vi "FiberMRI_Main_NI.vi"() -> ()   [LabVIEW 2010]
doc: "Acquisition software for combined single-photon fluorescence and fMRI experiments."
uses:
  typedefs/storage_parameters_cluster.ctl
  typedefs/experiment_mode_enum.ctl
  typedefs/stimulation_parameters.ctl
  typedefs/acquisition_parameters_NI_cluster.ctl
  typedefs/main_state_enum.ctl
  typedefs/control_daq_enum.ctl
  typedefs/control_display_enum.ctl
  typedefs/control_storage_enum.ctl
  typedefs/control_analysis_enum.ctl
  <vilib>/Utility/error.llb/DialogType.ctl
  typedefs/control_stim_enum.ctl
  typedefs/all_frontpanel_parameters_NI.ctl
  <vilib>/DAQmx/write.llb/DAQmx Write (Digital Bool 1Line 1Point).vi
  <vilib>/DAQmx/create/channels.llb/DAQmx Create Channel (DO-Digital Output).vi
  <vilib>/daqmx/miscellaneous.llb/DAQmx Fill In Error Info.vi
  globals/exit.vi
panel:
  in  "Acquisition parameters":T1={"Physical channels"="", "Shutter line"="", "Triggered?"=FALSE, "Sample rate"=1000.0, "Pixels to integrate"=10, "Effective data rate"=0.0, "Read chunk size"=100, "Samples to read"=2000, "Run mode"=enum."Continuously"} {"Pixels to integrate" min=1 step=1; "Sample rate" min=10.0 max=25000.0}
  out "Running":bool
  in  "Stimulation parameters":T2={"Physical channel"="Dev0/1stPortB/Do0", "Write chunk size"=1, "Sample rate"=1.0, "Stim onset"=0.0, "Stim frequency"=1.0, "ON time"=40.0, "OFF time"=120.0, "Repetitions"=1.0} {"Write chunk size" min=100 max=100000; "Sample rate" min=10.0 max=10000.0; "Repetitions" min=0.0 max=10.0 step=1.0; "OFF time" min=0.0 max=1000.0; "ON time" min=0.0 max=1000.0; "Stim onset" min=0.0 max=100.0; "Stim frequency" min=1.0 max=40.0 step=1.0}
  in  "Reset":bool
  in  "Shutter":bool
  in  "Experiment mode":T3
  in  "Storage parameters":T4
  in  "Run":bool
  in  "Quit":bool
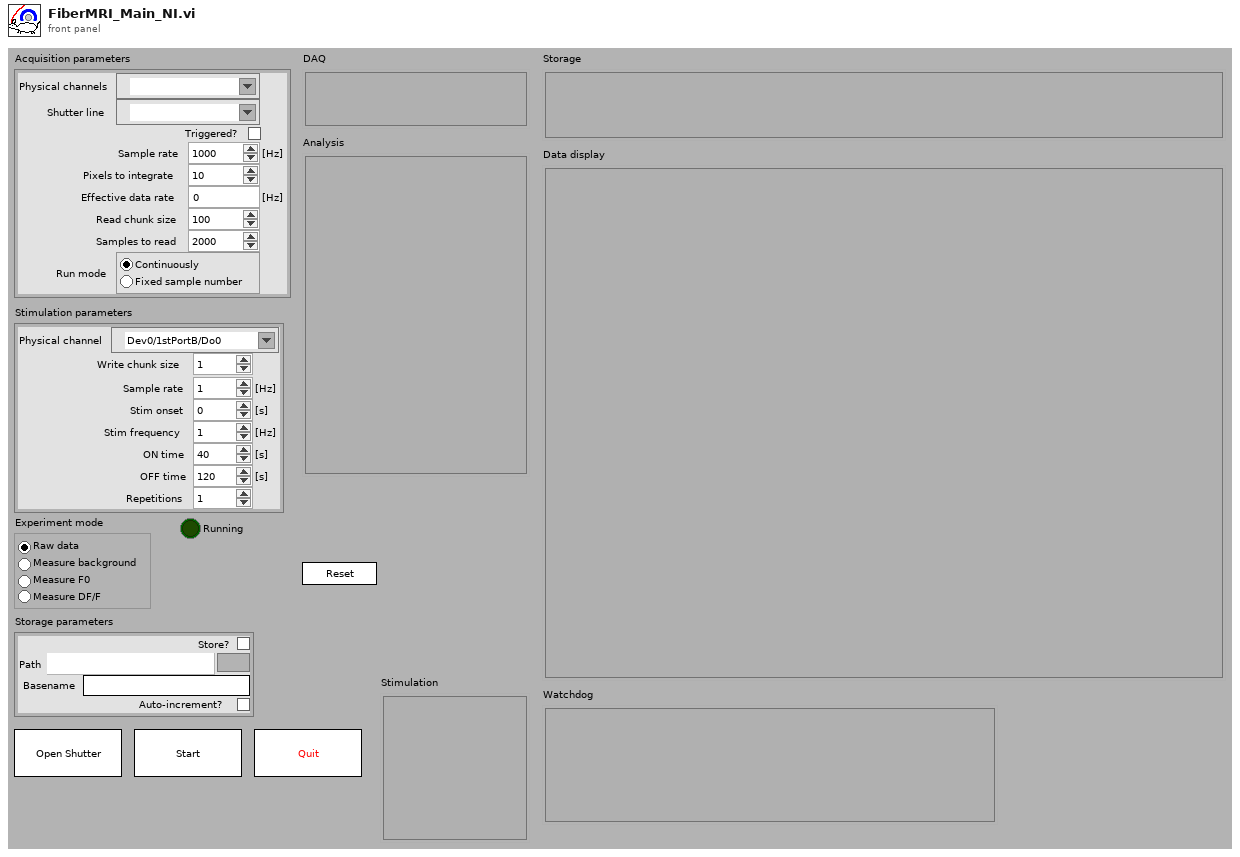
[diagram p1: front panel]
types:
  T1 = typedef "acquisition_parameters_NI_cluster.ctl" = cluster{"Physical channels":tag, "Shutter line":tag, "Triggered?":bool, "Sample rate":dbl, "Pixels to integrate":i32, "Effective data rate":dbl, "Read chunk size":i32, "Samples to read":i32, "Run mode":enum32{"Continuously", "Fixed sample number"}}
  T2 = typedef "stimulation_parameters.ctl" = cluster{"Physical channel":tag, "Write chunk size":i32, "Sample rate":dbl, "Stim onset":dbl, "Stim frequency":dbl, "ON time":dbl, "OFF time":dbl, "Repetitions":dbl}
  T3 = typedef "experiment_mode_enum.ctl" = enum32{"Raw data", "Measure background", "Measure F0", "Measure DF/F"}
  T4 = typedef "storage_parameters_cluster.ctl" = cluster{"Store?":bool, "Path":path, "Basename":string, "Auto-increment?":bool}
  T5 = typedef "all_frontpanel_parameters_NI.ctl" = cluster{"Acquisition parameters":T1, "Stimulation parameters":T2, "Experiment mode":T3, "Storage parameters":T4}
  T6 = typedef "DialogType.ctl" = u16
  T7 = typedef "main_state_enum.ctl" = enum16{"Init", "ParamsChanged", "Start", "Stop", "SetShutter", "Reset", "Save", "Quit"}
  T8 = cluster{"Control_DAQ_Queue":refnum<queue>, "Control_Storage_Queue":refnum<queue>, "Control_Display_Queue":refnum<queue>, "Control_Analysis_Queue":refnum<queue>, "Control_Stim_Queue":refnum<queue>}
  T9 = typedef "control_stim_enum.ctl" = enum16{"Init", "Stim", "Stop", "Quit"}
  T10 = cluster{"Control stim Enum":T9, "variant":variant}
  T11 = typedef "control_analysis_enum.ctl" = enum16{"Init", "Analyze", "Reset", "Stop", "Quit"}
  T12 = cluster{"Control Analysis Enum":T11, "variant":variant}
  T13 = typedef "control_display_enum.ctl" = enum16{"Init", "Display", "Quit"}
  T14 = cluster{"Control display enum":T13, "variant":variant}
  T15 = typedef "control_storage_enum.ctl" = enum16{"Init", "Discard", "Store", "Reset", "Stop", "Quit"}
  T16 = cluster{"Control storage enum":T15, "variant":variant}
  T17 = typedef "control_daq_enum.ctl" = enum16{"Init", "GetCont", "GetNoSamples", "Stop", "Quit"}
  T18 = cluster{"Control DAQ Enum":T17, "variant":variant}
  T19 = cluster{"Acquisition parameters":T1, "Stimulation parameters":T2}
  T20 = cluster{"Control DAQ Enum":T17, "Variant":variant}
  T21 = cluster{"Experiment mode":T3, "Pixels to integrate":i32, "#channels":i32, "Iteration":i32}
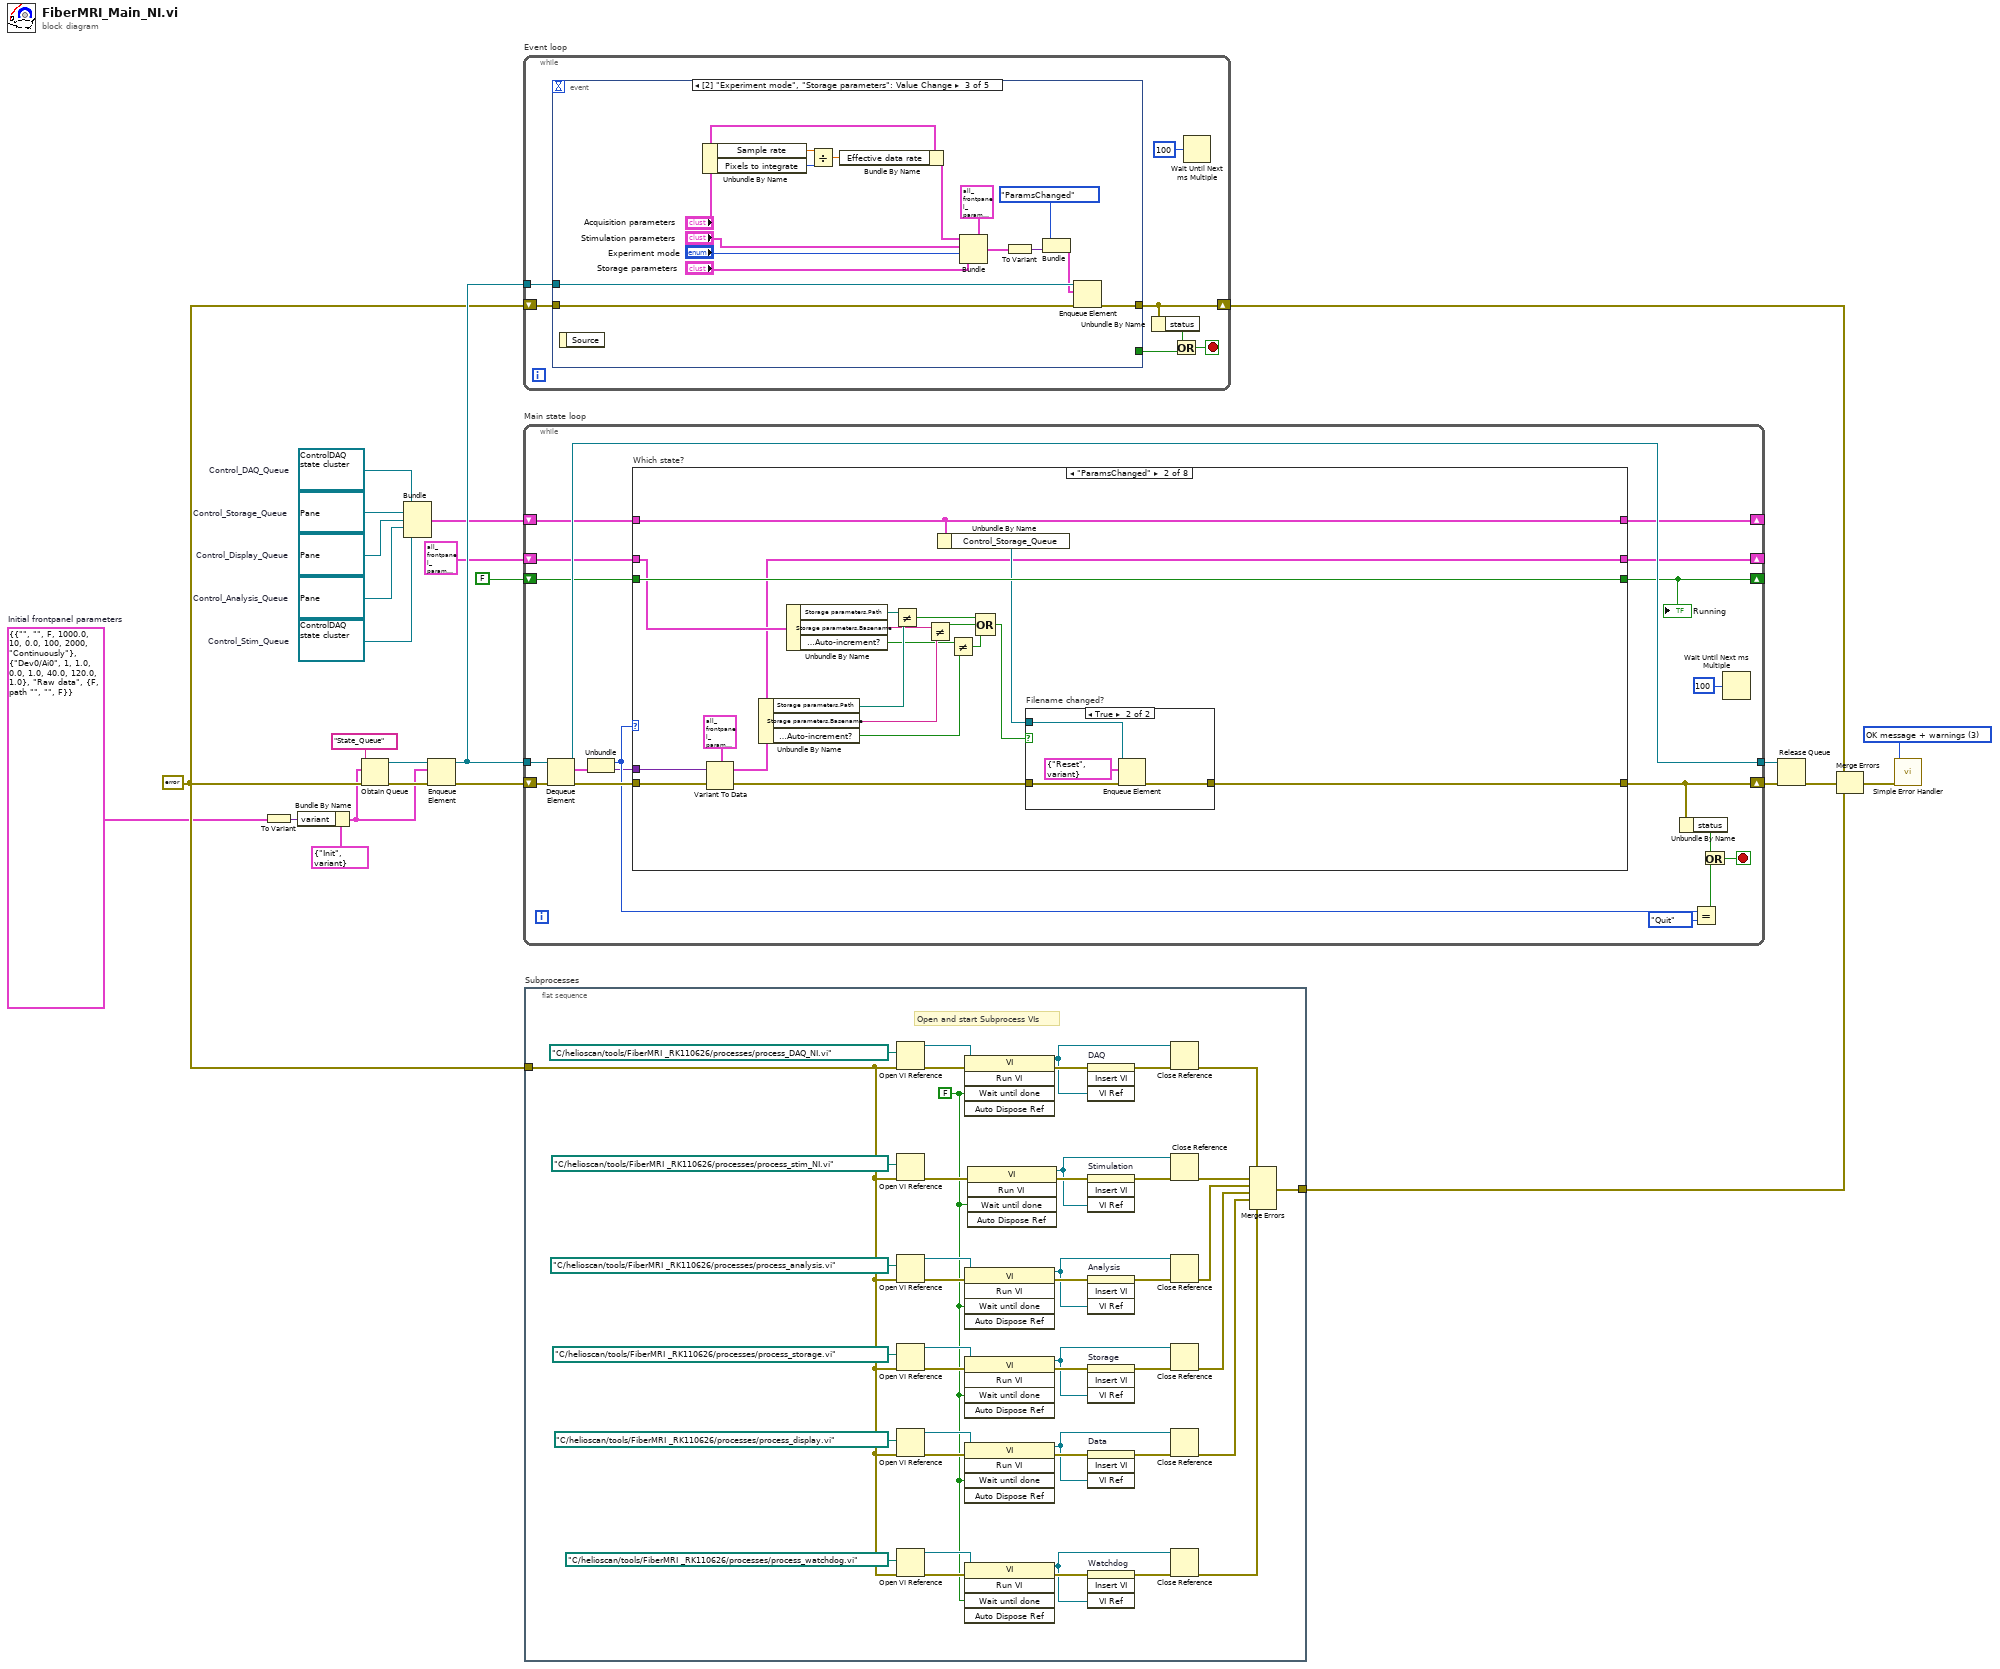
[diagram p0: block diagram]
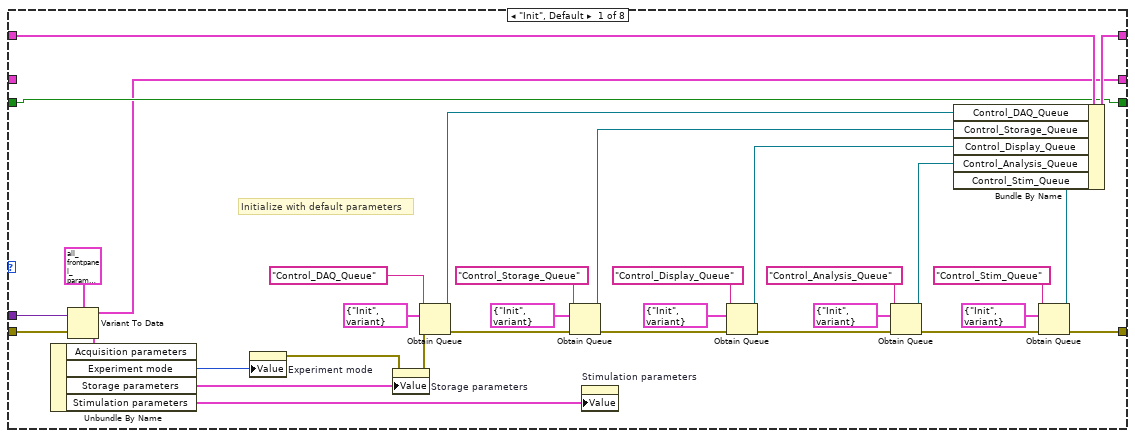
[diagram p2: hidden frame]
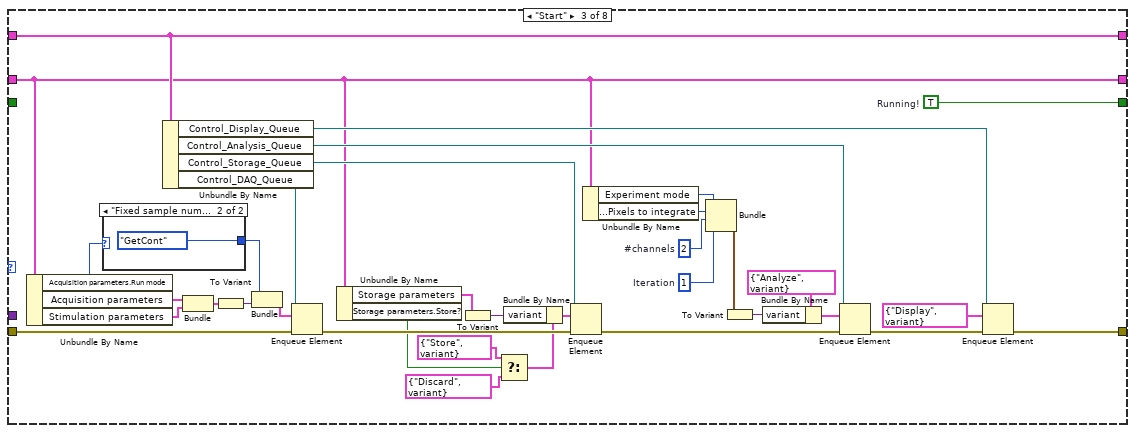
[diagram p4: hidden frame]
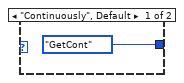
[diagram p5: hidden frame]
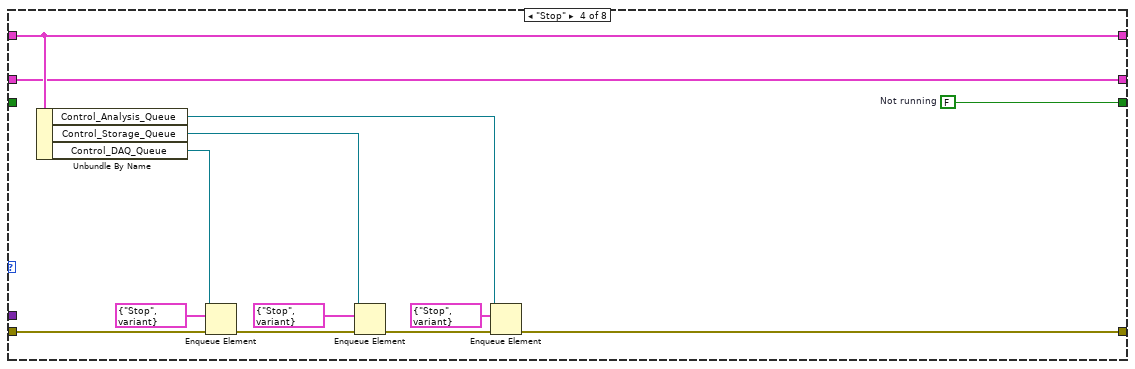
[diagram p6: hidden frame]
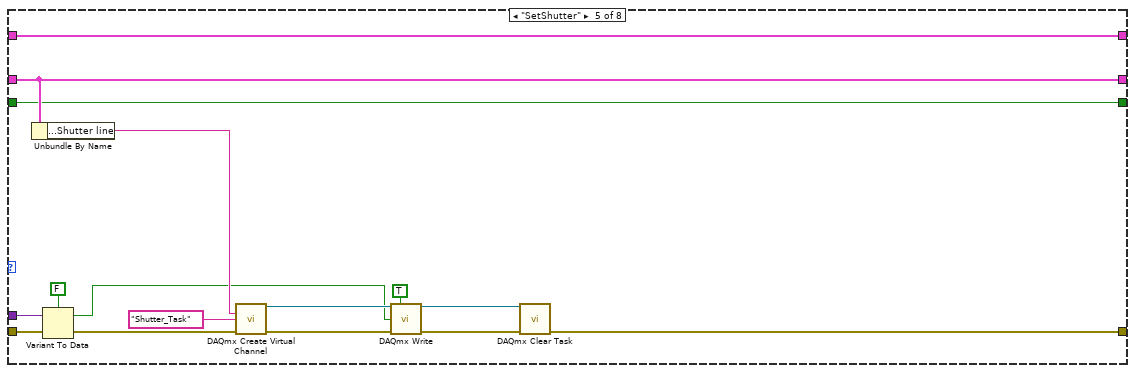
[diagram p7: hidden frame]
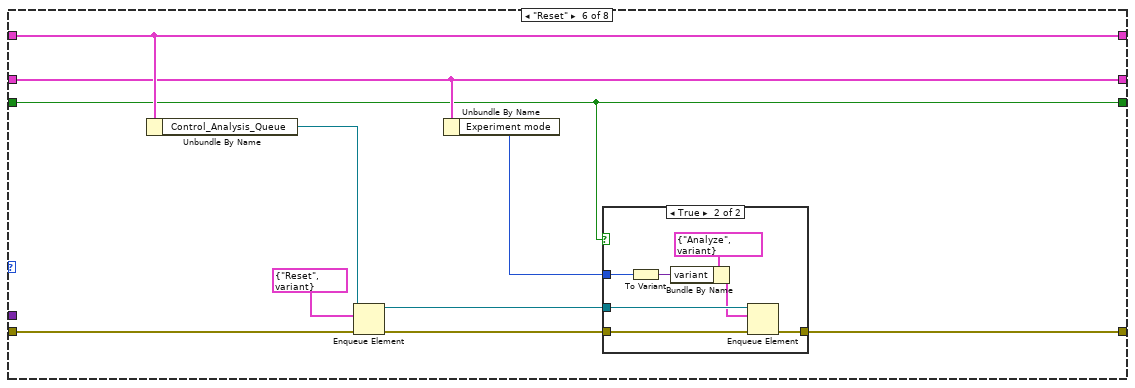
[diagram p8: hidden frame]
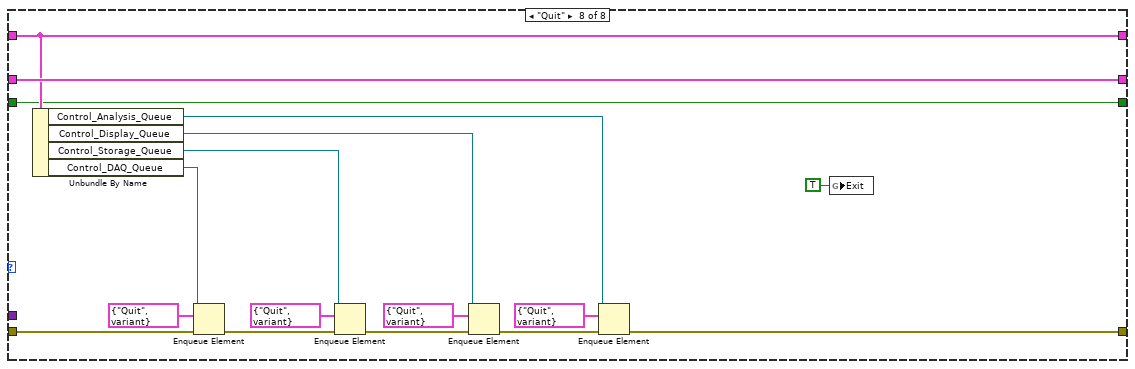
[diagram p11: hidden frame]
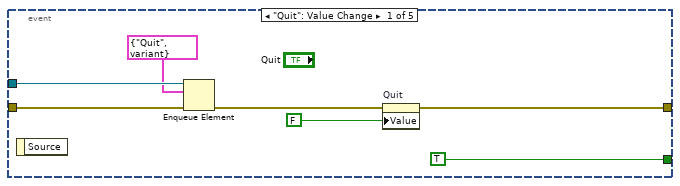
[diagram p12: hidden frame]
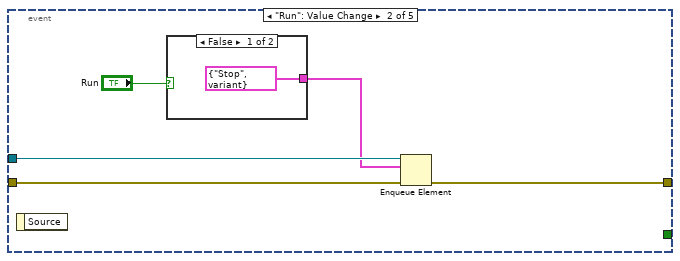
[diagram p13: hidden frame]
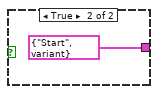
[diagram p14: hidden frame]
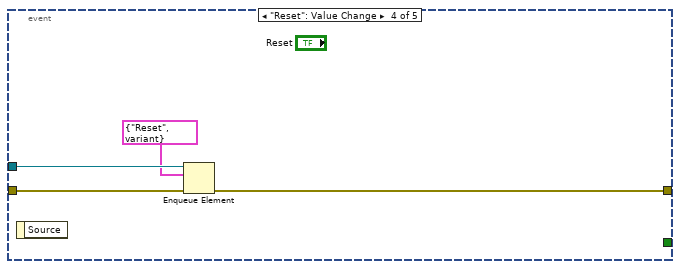
[diagram p15: hidden frame]
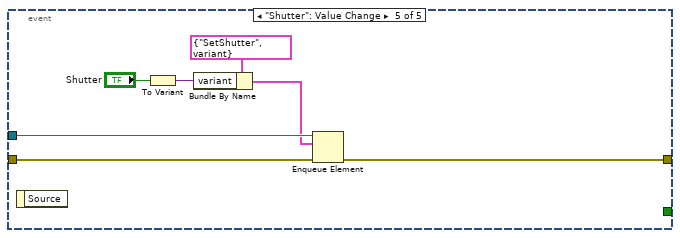
[diagram p16: hidden frame]
diagram:
  w2 = T5 {"Acquisition parameters"={"Physical channels"="", "Shutter line"="", "Triggered?"=FALSE, "Sample rate"=1000.0, "Pixels to integrate"=10, "Effective data rate"=0.0, "Read chunk size"=100, "Samples to read"=2000, "Run mode"=enum."Continuously"}, "Stimulation parameters"={"Physical channel"="Dev0/Ai0", "Write chunk size"=1, "Sample rate"=1.0, "Stim onset"=0.0, "Stim frequency"=1.0, "ON time"=40.0, "OFF time"=120.0, "Repetitions"=1.0}, "Experiment mode"=enum."Raw data", "Storage parameters"={"Store?"=FALSE, "Path"=path "", "Basename"="", "Auto-increment?"=FALSE}}  # Initial frontpanel parameters
  w3 = refnum<queue> refnum  # Control_Stim_Queue
  w13 = T6 3 items=["no dialog", "OK message", "continue or stop message", "OK message + warnings", "continue/stop + warnings"] ("type of dialog (OK msg:1)")
  w14 = refnum<queue> refnum  # Control_Analysis_Queue
  w15 = refnum<queue> refnum  # Control_Storage_Queue
  w16 = refnum<queue> refnum  # Control_Display_Queue
  w10 = errorcluster {"status"=FALSE, "code"=0, "source"=""} ("error out")
  w19 = refnum<queue> refnum  # Control_DAQ_Queue
  n1 = To Variant(anything=w2) -> (Variant=w5:variant)
  n2 = Bundle By Name(cluster=cluster{"State Enum":T7, "variant":variant} {"State Enum"=enum."Init", "variant"=variant}, "variant"=w5) -> (w4:cluster{"State Enum":T7, "variant":variant})
  n3 = Obtain Queue(name (unnamed)="State_Queue", element data type=w4, error in (no error)=w10) -> (queue out=w24:refnum<queue>, error out=w22:errorcluster)  [unwired: 2 in, 1 out]
  n4 = Bundle("Control_DAQ_Queue"=w19, "Control_Storage_Queue"=w15, "Control_Display_Queue"=w16, "Control_Analysis_Queue"=w14, "Control_Stim_Queue"=w3) -> (w18:T8)  [unwired: 1 in]
  n5 = Enqueue Element(queue=w24, element=w4, error in (no error)=w22) -> (queue out=w23:refnum<queue>, error out=w17:errorcluster)  [unwired: 1 in, 1 out]
  n6 = while "Event loop" {
    shift-right: [w28] -> w11
    shift-left: w10 -> [w31]
    tunnel: w23 -> [w32]
    stop <- w29 stop-if-true
    n7 = event shown="[2] \"Experiment mode\", \"Storage parameters\": Value Change" {
      selector: _ -> [_ _ _ _ _]
      dyn-events: _ -> [_ _ _ _ _]
      timeout: _ -> [_ _ _ _ _]
      tunnel: w32 -> [w38 w43 w62 w65 w72]
      tunnel: w31 -> [w39 w42 w47 w66 w73]
      tunnel: [w34 w40 w54 w64 w67] -> w28
      tunnel: [TRUE _ _ _ _] -> w30
      event "Quit": Value Change {
        n8 = event-data() -> ()  [unwired: 1 in, 1 out]
        n9 = Enqueue Element(queue=w38, element=cluster{"State Enum":T7, "variant":variant} {"State Enum"=enum."Quit", "variant"=variant}, error in (no error)=w39) -> (error out=w35:errorcluster)  [unwired: 1 in, 2 out]
        n10 = property on="Quit" class="Bool (strict)"(error in=w35, "Value"=FALSE) -> (error out=w34:errorcluster)  [unwired: 1 in, 1 out]
      }
      event "Run": Value Change {
        n11 = event-data() -> ()  [unwired: 1 in, 1 out]
        n12 = case shown="False" "Run" {
          tunnel: [cluster{"State Enum":T7, "variant":variant} {"State Enum"=enum."Stop", "variant"=variant} cluster{"State Enum":T7, "variant":variant} {"State Enum"=enum."Start", "variant"=variant}] -> w41
          frame False {
          }
          frame True {
          }
        }
        n13 = Enqueue Element(queue=w43, element=w41, error in (no error)=w42) -> (error out=w40:errorcluster)  [unwired: 1 in, 2 out]
      }
      event Value Change {
        n14 = event-data() -> ()  [unwired: 1 in, 1 out]
        n15 = Unbundle By Name("Acquisition parameters") -> ("Sample rate"=w56:dbl, "Pixels to integrate"=w57:i32)
        n16 = Divide(x=w56, y=w57) -> (x/y=w55:dbl)
        n17 = Bundle By Name(cluster="Acquisition parameters", "Effective data rate"=w55) -> (w53:T1)
        n18 = Bundle(cluster=T5 {"Acquisition parameters"={"Physical channels"="", "Shutter line"="", "Triggered?"=FALSE, "Sample rate"=1000.0, "Pixels to integrate"=10, "Effective data rate"=0.0, "Read chunk size"=100, "Samples to read"=2000, "Run mode"=enum."Continuously"}, "Stimulation parameters"={"Physical channel"="Dev0/Ai0", "Write chunk size"=1, "Sample rate"=1.0, "Stim onset"=0.0, "Stim frequency"=1.0, "ON time"=40.0, "OFF time"=120.0, "Repetitions"=1.0}, "Experiment mode"=enum."Raw data", "Storage parameters"={"Store?"=FALSE, "Path"=path "", "Basename"="", "Auto-increment?"=FALSE}} ("All frontpanel parameters"), "Acquisition parameters"=w53, "Stimulation parameters"="Stimulation parameters", "Experiment mode"="Experiment mode", "Storage parameters"="Storage parameters") -> (w58:T5)
        n19 = To Variant(anything=w58) -> (Variant=w61:variant)
        n20 = Bundle("State Enum"=main_state_enum."ParamsChanged", "Variant"=w61) -> (w59:cluster{"State Enum":T7, "Variant":variant})  [unwired: 1 in]
        n21 = Enqueue Element(queue=w62, element=w59, error in (no error)=w47) -> (error out=w54:errorcluster)  [unwired: 1 in, 2 out]
      }
      event "Reset": Value Change {
        n22 = event-data() -> ()  [unwired: 1 in, 1 out]
        n23 = Enqueue Element(queue=w65, element=cluster{"State Enum":T7, "variant":variant} {"State Enum"=enum."Reset", "variant"=variant}, error in (no error)=w66) -> (error out=w64:errorcluster)  [unwired: 1 in, 2 out]
      }
      event "Shutter": Value Change {
        n24 = event-data() -> ()  [unwired: 1 in, 1 out]
        n25 = To Variant(anything="Shutter") -> (Variant=w70:variant)
        n26 = Bundle By Name(cluster=cluster{"State Enum":T7, "variant":variant} {"State Enum"=enum."SetShutter", "variant"=variant} ("element"), "variant"=w70) -> (w68:cluster{"State Enum":T7, "variant":variant})
        n27 = Enqueue Element(queue=w72, element=w68, error in (no error)=w73) -> (error out=w67:errorcluster)  [unwired: 1 in, 2 out]
      }
    }
    n28 = Unbundle By Name(w28) -> ("status"=w27:bool)
    n29 = Or(x=w27, y=w30) -> (x .or. y?=w29:bool)
    n30 = Wait Until Next ms Multiple(millisecond multiple=u32 100) -> ()  [unwired: 1 out]
  }
  n31 = while "Main state loop" {
    shift-right: [w80] -> w25
    shift-left: w17 -> [w90]
    shift-right: [w84] -> _
    shift-left: T5 {"Acquisition parameters"={"Physical channels"="", "Shutter line"="", "Triggered?"=FALSE, "Sample rate"=1000.0, "Pixels to integrate"=10, "Effective data rate"=0.0, "Read chunk size"=100, "Samples to read"=2000, "Run mode"=enum."Continuously"}, "Stimulation parameters"={"Physical channel"="Dev0/Ai0", "Write chunk size"=1, "Sample rate"=1.0, "Stim onset"=0.0, "Stim frequency"=1.0, "ON time"=40.0, "OFF time"=120.0, "Repetitions"=1.0}, "Experiment mode"=enum."Raw data", "Storage parameters"={"Store?"=FALSE, "Path"=path "", "Basename"="", "Auto-increment?"=FALSE}} ("Initial frontpanel parameters") -> [w83]
    tunnel: w23 -> [w92]
    tunnel: [w91] -> w21
    shift-right: [w81] -> _
    shift-left: w18 -> [w82]
    shift-right: [w75] -> _
    shift-left: FALSE -> [w76]
    stop <- w77 stop-if-true
    n32 = Dequeue Element(queue=w92, error in (no error)=w90) -> (queue out=w91:refnum<queue>, element=w87:cluster{"State Enum":T7, "variant":variant}, error out=w89:errorcluster)  [unwired: 1 in, 1 out]
    n33 = Unbundle(w87) -> ("State Enum"=w86:T7, "variant"=w85:variant)
    n34 = case "Which state?" shown="\"ParamsChanged\"" w86 {
      tunnel: w89 -> [w101 w143 w184 w199 w213 w224 w237 w254]
      tunnel: [w97 w127 w175 w189 w200 w219 w237 w242] -> w80
      tunnel: w85 -> [w99 w144 _ _ w212 _ _ _]
      tunnel: [w100 w126 w165 w188 w214 w221 w236 w253] -> w84
      tunnel: w83 -> [_ w141 w165 w188 w214 w221 w236 w253]
      tunnel: w82 -> [w120 w130 w179 w197 w215 w225 w235 w251]
      tunnel: [w119 w130 w179 w197 w215 w225 w235 w251] -> w81
      tunnel: w76 -> [w107 w142 _ _ w210 w216 w234 w239]
      tunnel: [w107 w142 w166 w187 w210 w216 w234 w239] -> w75
      frame "Init", Default {
        # "Initialize with default parameters"
        n35 = Variant To Data(error in=w101, Variant=w99, type=T5 {"Acquisition parameters"={"Physical channels"="", "Shutter line"="", "Triggered?"=FALSE, "Sample rate"=1000.0, "Pixels to integrate"=10, "Effective data rate"=0.0, "Read chunk size"=100, "Samples to read"=2000, "Run mode"=enum."Continuously"}, "Stimulation parameters"={"Physical channel"="Dev0/Ai0", "Write chunk size"=1, "Sample rate"=1.0, "Stim onset"=0.0, "Stim frequency"=1.0, "ON time"=40.0, "OFF time"=120.0, "Repetitions"=1.0}, "Experiment mode"=enum."Raw data", "Storage parameters"={"Store?"=FALSE, "Path"=path "", "Basename"="", "Auto-increment?"=FALSE}} ("Initial frontpanel parameters")) -> (data=w100:T5)  [unwired: 1 out]
        n36 = Unbundle By Name(w100) -> ("Experiment mode"=w106:T3, "Storage parameters"=w103:T4, "Stimulation parameters"=w102:T2)  [unwired: 1 out]
        n37 = property on="Experiment mode" class="RadioBtnsControl (strict)"("Value"=w106) -> (error out=w105:errorcluster)  [unwired: 2 in, 1 out]
        n38 = property on="Storage parameters" class="Clust (strict)"(error in=w105, "Value"=w103) -> (error out=w104:errorcluster)  [unwired: 1 in, 1 out]
        n39 = Obtain Queue(name (unnamed)="Control_DAQ_Queue", element data type=T18 {"Control DAQ Enum"=enum."Init", "variant"=variant} ("ControlDAQ state cluster"), error in (no error)=w104) -> (queue out=w118:refnum<queue>, error out=w116:errorcluster)  [unwired: 2 in, 1 out]
        n40 = Obtain Queue(name (unnamed)="Control_Storage_Queue", element data type=T16 {"Control storage enum"=enum."Init", "variant"=variant}, error in (no error)=w116) -> (queue out=w117:refnum<queue>, error out=w115:errorcluster)  [unwired: 2 in, 1 out]
        n41 = property on="Stimulation parameters" class="Clust (strict)"("Value"=w102) -> ()  [unwired: 2 in, 2 out]
        n42 = Obtain Queue(name (unnamed)="Control_Display_Queue", element data type=T14 {"Control display enum"=enum."Init", "variant"=variant}, error in (no error)=w115) -> (queue out=w112:refnum<queue>, error out=w111:errorcluster)  [unwired: 2 in, 1 out]
        n43 = Obtain Queue(name (unnamed)="Control_Analysis_Queue", element data type=T12 {"Control Analysis Enum"=enum."Init", "variant"=variant}, error in (no error)=w111) -> (queue out=w108:refnum<queue>, error out=w98:errorcluster)  [unwired: 2 in, 1 out]
        n44 = Obtain Queue(name (unnamed)="Control_Stim_Queue", element data type=T10 {"Control stim Enum"=enum."Init", "variant"=variant} ("ControlDAQ state cluster"), error in (no error)=w98) -> (queue out=w94:refnum<queue>, error out=w97:errorcluster)  [unwired: 2 in, 1 out]
        n45 = Bundle By Name(cluster=w120, "Control_DAQ_Queue"=w118, "Control_Storage_Queue"=w117, "Control_Display_Queue"=w112, "Control_Analysis_Queue"=w108, "Control_Stim_Queue"=w94) -> (w119:T8)
      }
      frame "ParamsChanged" {
        n46 = Variant To Data(error in=w143, Variant=w144, type=T5 {"Acquisition parameters"={"Physical channels"="", "Shutter line"="", "Triggered?"=FALSE, "Sample rate"=1000.0, "Pixels to integrate"=10, "Effective data rate"=0.0, "Read chunk size"=100, "Samples to read"=2000, "Run mode"=enum."Continuously"}, "Stimulation parameters"={"Physical channel"="Dev0/Ai0", "Write chunk size"=1, "Sample rate"=1.0, "Stim onset"=0.0, "Stim frequency"=1.0, "ON time"=40.0, "OFF time"=120.0, "Repetitions"=1.0}, "Experiment mode"=enum."Raw data", "Storage parameters"={"Store?"=FALSE, "Path"=path "", "Basename"="", "Auto-increment?"=FALSE}} ("Initial frontpanel parameters")) -> (error out=w128:errorcluster, data=w126:T5)
        n47 = Unbundle By Name(w126) -> ("Storage parameters.Path"=w139:path, "Storage parameters.Basename"=w137:string, "Storage parameters.Auto-increment?"=w135:bool)
        n48 = Unbundle By Name(w141) -> ("Storage parameters.Path"=w140:path, "Storage parameters.Basename"=w138:string, "Storage parameters.Auto-increment?"=w136:bool)
        n49 = Not Equal?(x=w140, y=w139) -> (x != y?=w134:bool)
        n50 = Not Equal?(x=w138, y=w137) -> (x != y?=w133:bool)
        n51 = Unbundle By Name(w130) -> ("Control_Storage_Queue"=w129:refnum<queue>)
        n52 = Not Equal?(x=w136, y=w135) -> (x != y?=w132:bool)
        n53 = Compound Arithmetic op=OR(w134, w133, w132) -> (w131:bool)
        n54 = case "Filename changed?" shown="True" w131 {
          tunnel: w129 -> [_ w149]
          tunnel: w128 -> [w145 w147]
          tunnel: [w145 w146] -> w127
          frame False {
          }
          frame True {
            n55 = Enqueue Element(queue=w149, element=T16 {"Control storage enum"=enum."Reset", "variant"=variant}, error in (no error)=w147) -> (error out=w146:errorcluster)  [unwired: 1 in, 2 out]
          }
        }
      }
      frame "Start" {
        w150 = 1  # Iteration
        w151 = 2  # #channels
        w166 = TRUE  # Running!
        n56 = Unbundle By Name(w165) -> ("Acquisition parameters.Run mode"=w181:enum32{"Continuously", "Fixed sample number"}, "Acquisition parameters"=w160:T1, "Stimulation parameters"=w159:T2)
        n57 = case shown="\"Fixed sample number\"" w181 {
          tunnel: [control_daq_enum."GetCont" ("Control DAQ Enum") control_daq_enum."GetCont" ("Control DAQ Enum")] -> w180
          frame "Continuously", Default {
          }
          frame "Fixed sample number" {
          }
        }
        n58 = Unbundle By Name(w179) -> ("Control_Display_Queue"=w173:refnum<queue>, "Control_Analysis_Queue"=w170:refnum<queue>, "Control_Storage_Queue"=w176:refnum<queue>, "Control_DAQ_Queue"=w178:refnum<queue>)
        n59 = Bundle("Acquisition parameters"=w160, "Stimulation parameters"=w159) -> (w158:T19)  [unwired: 1 in]
        n60 = To Variant(anything=w158) -> (Variant=w183:variant)
        n61 = Bundle("Control DAQ Enum"=w180, "Variant"=w183) -> (w182:T20)  [unwired: 1 in]
        n62 = Enqueue Element(queue=w178, element=w182, error in (no error)=w184) -> (error out=w177:errorcluster)  [unwired: 1 in, 2 out]
        n63 = Unbundle By Name(w165) -> ("Storage parameters"=w161:T4, "Storage parameters.Store?"=w156:bool)
        n64 = To Variant(anything=w161) -> (Variant=w157:variant)
        n65 = Select(t=T16 {"Control storage enum"=enum."Store", "variant"=variant} ("element"), s=w156, f=T16 {"Control storage enum"=enum."Discard", "variant"=variant} ("element")) -> (s? t:f=w153:T16)
        n66 = Bundle By Name(cluster=w153, "variant"=w157) -> (w152:T16)
        n67 = Enqueue Element(queue=w176, element=w152, error in (no error)=w177) -> (error out=w172:errorcluster)  [unwired: 1 in, 2 out]
        n68 = Unbundle By Name(w165) -> ("Experiment mode"=w164:T3, "Acquisition parameters.Pixels to integrate"=w163:i32)
        n69 = Bundle("Experiment mode"=w164, "Pixels to integrate"=w163, "#channels"=w151, "Iteration"=w150) -> (w162:T21)  [unwired: 1 in]
        n70 = To Variant(anything=w162) -> (Variant=w169:variant)
        n71 = Bundle By Name(cluster=T12 {"Control Analysis Enum"=enum."Analyze", "variant"=variant} ("element"), "variant"=w169) -> (w167:T12)
        n72 = Enqueue Element(queue=w170, element=w167, error in (no error)=w172) -> (error out=w171:errorcluster)  [unwired: 1 in, 2 out]
        n73 = Enqueue Element(queue=w173, element=T14 {"Control display enum"=enum."Display", "variant"=variant}, error in (no error)=w171) -> (error out=w175:errorcluster)  [unwired: 1 in, 2 out]
      }
      frame "Stop" {
        w187 = FALSE  # Not running
        n74 = Unbundle By Name(w197) -> ("Control_Analysis_Queue"=w191:refnum<queue>, "Control_Storage_Queue"=w194:refnum<queue>, "Control_DAQ_Queue"=w196:refnum<queue>)
        n75 = Enqueue Element(queue=w196, element=T18 {"Control DAQ Enum"=enum."Stop", "variant"=variant}, error in (no error)=w199) -> (error out=w195:errorcluster)  [unwired: 1 in, 2 out]
        n76 = Enqueue Element(queue=w194, element=T16 {"Control storage enum"=enum."Stop", "variant"=variant}, error in (no error)=w195) -> (error out=w192:errorcluster)  [unwired: 1 in, 2 out]
        n77 = Enqueue Element(queue=w191, element=T12 {"Control Analysis Enum"=enum."Stop", "variant"=variant}, error in (no error)=w192) -> (error out=w189:errorcluster)  [unwired: 1 in, 2 out]
      }
      frame "SetShutter" {
        n78 = Unbundle By Name(w214) -> ("Acquisition parameters.Shutter line"=w208:tag)
        n79 = Variant To Data(error in=w213, Variant=w212, type=FALSE) -> (error out=w209:errorcluster, data=w204:bool)
        n80 = call-poly <vilib>:"DAQmx Create Virtual Channel.vi"("lines"=w208, "name to assign"="Shutter_Task", "error in"=w209) -> ("task out"=w205:refnum<k21>, "error out"=w206:errorcluster)  [unwired: 11 in]
        n81 = call-poly <vilib>:"DAQmx Write.vi"("task/channels in"=w205, "auto start"=TRUE, "data"=w204, "error in"=w206) -> ("task out"=w201:refnum<k21>, "error out"=w202:errorcluster)  [unwired: 9 in, 1 out]
        n82 = call <vilib>:"DAQmx Clear Task.vi"("task in"=w201, "error in"=w202) -> ("error out"=w200:errorcluster)  [unwired: 13 in]
      }
      frame "Reset" {
        n83 = Unbundle By Name(w225) -> ("Control_Analysis_Queue"=w223:refnum<queue>)
        n84 = Enqueue Element(queue=w223, element=T12 {"Control Analysis Enum"=enum."Reset", "variant"=variant}, error in (no error)=w224) -> (queue out=w218:refnum<queue>, error out=w220:errorcluster)  [unwired: 1 in, 1 out]
        n85 = Unbundle By Name(w221) -> ("Experiment mode"=w217:T3)
        n86 = case shown="True" w216 {
          tunnel: [w226 w232] -> w219
          tunnel: w220 -> [w226 w233]
          tunnel: w218 -> [_ w231]
          tunnel: w217 -> [_ w230]
          frame False {
          }
          frame True {
            n87 = To Variant(anything=w230) -> (Variant=w227:variant)
            n88 = Bundle By Name(cluster=T12 {"Control Analysis Enum"=enum."Analyze", "variant"=variant} ("element"), "variant"=w227) -> (w228:T12)
            n89 = Enqueue Element(queue=w231, element=w228, error in (no error)=w233) -> (error out=w232:errorcluster)  [unwired: 1 in, 2 out]
          }
        }
      }
      frame "Save" {
      }
      frame "Quit" {
        n90 = Unbundle By Name(w251) -> ("Control_Analysis_Queue"=w241:refnum<queue>, "Control_Display_Queue"=w245:refnum<queue>, "Control_Storage_Queue"=w248:refnum<queue>, "Control_DAQ_Queue"=w250:refnum<queue>)
        n91 = Enqueue Element(queue=w250, element=T18 {"Control DAQ Enum"=enum."Quit", "variant"=variant} ("ControlDAQ state cluster"), error in (no error)=w254) -> (error out=w249:errorcluster)  [unwired: 1 in, 2 out]
        n92 = Enqueue Element(queue=w248, element=T16 {"Control storage enum"=enum."Quit", "variant"=variant}, error in (no error)=w249) -> (error out=w246:errorcluster)  [unwired: 1 in, 2 out]
        n93 = Enqueue Element(queue=w245, element=T14 {"Control display enum"=enum."Quit", "variant"=variant}, error in (no error)=w246) -> (error out=w243:errorcluster)  [unwired: 1 in, 2 out]
        n94 = Enqueue Element(queue=w241, element=T12 {"Control Analysis Enum"=enum."Quit", "variant"=variant}, error in (no error)=w243) -> (error out=w242:errorcluster)  [unwired: 1 in, 2 out]
        n95 = global write "exit.vi" "Exit"(TRUE ("Exit")) -> ()
      }
    }
    "Running" <- w75
    n96 = Unbundle By Name(w80) -> ("status"=w79:bool)
    n97 = Equal?(x=w86, y=main_state_enum."Quit") -> (x = y?=w78:bool)
    n98 = Or(x=w79, y=w78) -> (x .or. y?=w77:bool)
    n99 = Wait Until Next ms Multiple(millisecond multiple=u32 100) -> ()  [unwired: 1 out]
  }
  n100 = flat-sequence "Subprocesses" {
    tunnel: w10 -> [w261]
    tunnel: [w278] -> w7
    frame #0 {
      w260 = FALSE ("Wait Until Done")
      # "Open and start Subprocess VIs"
      n101 = Open VI Reference(vi path=path "C:/helioscan/tools/FiberMRI _RK110626/processes/process_DAQ_NI.vi", error in (no error)=w261) -> (vi reference=w293:refnum<vi>, error out=w294:errorcluster)  [unwired: 4 in]
      n102 = Open VI Reference(vi path=path "C:/helioscan/tools/FiberMRI _RK110626/processes/process_stim_NI.vi", error in (no error)=w261) -> (error out=w262:errorcluster)  [unwired: 4 in, 1 out]
      n103 = Open VI Reference(vi path=path "C:/helioscan/tools/FiberMRI _RK110626/processes/process_analysis.vi", error in (no error)=w261) -> (vi reference=w291:refnum<vi>, error out=w292:errorcluster)  [unwired: 4 in]
      n104 = Open VI Reference(vi path=path "C:/helioscan/tools/FiberMRI _RK110626/processes/process_storage.vi", error in (no error)=w261) -> (vi reference=w289:refnum<vi>, error out=w290:errorcluster)  [unwired: 4 in]
      n105 = Open VI Reference(vi path=path "C:/helioscan/tools/FiberMRI _RK110626/processes/process_display.vi", error in (no error)=w261) -> (vi reference=w287:refnum<vi>, error out=w288:errorcluster)  [unwired: 4 in]
      n106 = Open VI Reference(vi path=path "C:/helioscan/tools/FiberMRI _RK110626/processes/process_watchdog.vi", error in (no error)=w261) -> (vi reference=w275:refnum<vi>, error out=w277:errorcluster)  [unwired: 4 in]
      n107 = invoke class="VI" method="Run VI"(reference=w293, error in=w294, "Wait until done"=w260) -> (reference out=w268:refnum<vi>, error out=w270:errorcluster)  [unwired: 2 in, 3 out]
      n108 = invoke class="VI" method="Run VI"(reference=w291, error in=w292, "Wait until done"=w260) -> (reference out=w283:refnum<vi>, error out=w286:errorcluster)  [unwired: 2 in, 3 out]
      n109 = invoke class="VI" method="Run VI"(reference=w289, error in=w290, "Wait until done"=w260) -> (reference out=w264:refnum<vi>, error out=w267:errorcluster)  [unwired: 2 in, 3 out]
      n110 = invoke class="VI" method="Run VI"(reference=w287, error in=w288, "Wait until done"=w260) -> (reference out=w281:refnum<vi>, error out=w285:errorcluster)  [unwired: 2 in, 3 out]
      n111 = invoke class="VI" method="Run VI"(reference=w275, error in=w277, "Wait until done"=w260) -> (reference out=w272:refnum<vi>, error out=w274:errorcluster)  [unwired: 2 in, 3 out]
      n112 = invoke class="VI" method="Run VI"(error in=w262, "Wait until done"=w260) -> (reference out=w257:refnum<vi>, error out=w259:errorcluster)  [unwired: 3 in, 3 out]
      n113 = invoke on="DAQ" class="SubPanel" method="Insert VI"(error in=w270, "VI Ref"=w268) -> (error out=w269:errorcluster)  [unwired: 2 in, 3 out]
      n114 = invoke on="Stimulation" class="SubPanel" method="Insert VI"(error in=w259, "VI Ref"=w257) -> (error out=w258:errorcluster)  [unwired: 2 in, 3 out]
      n115 = invoke on="Analysis" class="SubPanel" method="Insert VI"(error in=w286, "VI Ref"=w283) -> (error out=w284:errorcluster)  [unwired: 2 in, 3 out]
      n116 = invoke on="Storage" class="SubPanel" method="Insert VI"(error in=w267, "VI Ref"=w264) -> (error out=w266:errorcluster)  [unwired: 2 in, 3 out]
      n117 = invoke on="Data" class="SubPanel" method="Insert VI"(error in=w285, "VI Ref"=w281) -> (error out=w282:errorcluster)  [unwired: 2 in, 3 out]
      n118 = invoke on="Watchdog" class="SubPanel" method="Insert VI"(error in=w274, "VI Ref"=w272) -> (error out=w273:errorcluster)  [unwired: 2 in, 3 out]
      n119 = Close Reference(reference=w268, error in (no error)=w269) -> (error out=w256:errorcluster)
      n120 = Close Reference(reference=w257, error in (no error)=w258) -> (error out=w255:errorcluster)
      n121 = Close Reference(reference=w283, error in (no error)=w284) -> (error out=w279:errorcluster)
      n122 = Close Reference(reference=w264, error in (no error)=w266) -> (error out=w265:errorcluster)
      n123 = Close Reference(reference=w281, error in (no error)=w282) -> (error out=w280:errorcluster)
      n124 = Close Reference(reference=w272, error in (no error)=w273) -> (error out=w271:errorcluster)
      n125 = Merge Errors(w256, w255, w279, w265, w280, w271) -> (w278:errorcluster)
    }
  }
  n126 = Release Queue(queue=w21, error in (no error)=w25) -> (error out=w9:errorcluster)  [unwired: 1 in, 2 out]
  n127 = Merge Errors(w11, w9, w7) -> (w12:errorcluster)
  n128 = call <vilib>:"Simple Error Handler.vi"("type of dialog (OK msg:1)"=w13, "error in (no error)"=w12) -> ()  [unwired: 3 in, 5 out]
